vi "CSM Tool Name from VI.vi"(11 "VI Path":path) -> (3 "ToolName":string)   [LabVIEW 2017, in "CSM DebugTool Dialog.lvlib"]
uses:
  CSM DebugTool Dialog.lvlib
  _Shared/CSM Shared.lvlib
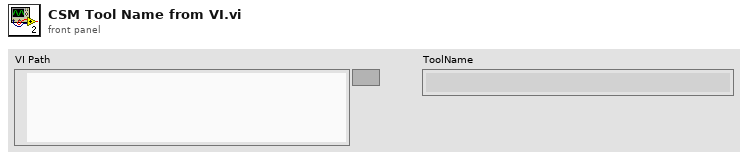
[diagram p1: front panel]
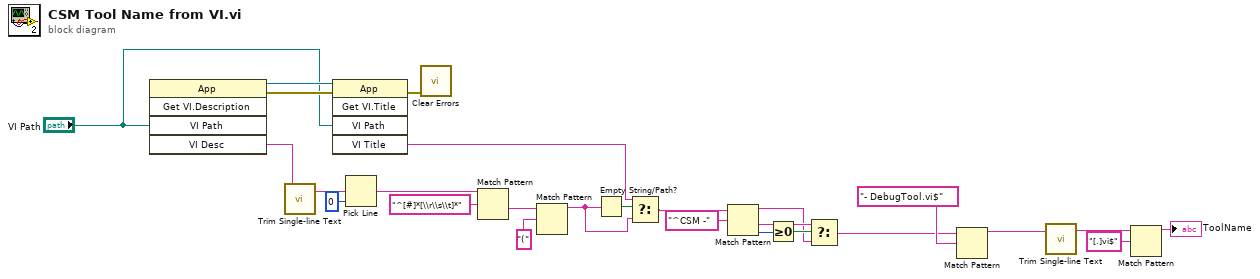
[diagram p0: block diagram]
diagram:
  n1 = invoke class="App" method="Get VI.Description"("VI Path"="VI Path") -> (reference out=w25:refnum<vi>, error out=w26:errorcluster, "VI Desc"=w23:string)  [unwired: 4 in, 2 out]
  n2 = call "Trim Single-line Text.vi"("single-line text"=w23) -> ("trimed text"=w22:string)  [unwired: 2 in]
  n3 = invoke class="App" method="Get VI.Title"(reference=w25, error in=w26, "VI Path"="VI Path") -> (error out=w3:errorcluster, "VI Title"=w14:string)  [unwired: 2 in, 3 out]
  n4 = Pick Line(multi-line string=w22, line index=0) -> (output string=w20:string)  [unwired: 1 in]
  n5 = call <vilib>:"Clear Errors.vi"("error in (no error)"=w3) -> ()  [unwired: 5 in, 2 out]
  n6 = Match Pattern(string=w20, regular expression="^[#]*[\\r\\s\\t]*") -> (after substring=w18:string)  [unwired: 1 in, 3 out]
  n7 = Match Pattern(string=w18, regular expression="(") -> (before substring=w13:string)  [unwired: 1 in, 3 out]
  n8 = Empty String/Path?(string/path=w13) -> (empty?=w16:bool)
  n9 = Select(t=w14, s=w16, f=w13) -> (s? t:f=w6:string)
  n10 = Match Pattern(string=w6, regular expression="^CSM -") -> (before substring=w7:string, after substring=w8:string, offset past match=w10:i32)  [unwired: 1 in, 1 out]
  n11 = Greater Or Equal To 0?(x=w10) -> (x >= 0?=w9:bool)
  n12 = Select(t=w8, s=w9, f=w7) -> (s? t:f=w2:string)
  n13 = Match Pattern(string=w2, regular expression="- DebugTool.vi$") -> (before substring=w1:string)  [unwired: 1 in, 3 out]
  n14 = call "Trim Single-line Text.vi"("single-line text"=w1) -> ("trimed text"=w5:string)  [unwired: 2 in]
  n15 = Match Pattern(string=w5, regular expression="[.]vi$") -> (before substring=→"ToolName":string)  [unwired: 1 in, 3 out]
